vi "CSMStandApp.vi"() -> ()   [LabVIEW 2020]
doc: "------------- lvcsm -------------\n[CSMStates]\nItem 0 = \"Event Structure\"\nItem 1 = \"Idle\"\nItem 2 = \"CSM Documentation\"\nItem 3 = \"VI Reference\"\nItem 4 = \"Error Handler\"\nItem 5 = \"Critical Error\"\nItem 6 = \"Target Timeout Error\"\nItem 7 = \"Target Error\"\nItem 8 = \"Async Response\"\nItem 9 = \"Response\"\nItem 10 = \"Async Message Posted\"\nItem 11 = \"Initialize Core Data\"\nItem 12 = \"Exit\"\nItem 13 = \"Data: Initialize\"\nItem 14 = \"Data: Get Configuration\"\nItem 15 = \"Data: Get Internal Data\"\nItem 16 = \"Data: Set Configuration\"\nItem 17 = \"Data: Cleanup\"\nItem 18 = \"Events: Register\"\nItem 19 = \"Events: Unregister\"\nItem 20 = \"UI: Initialize\"\nItem 21 = \"UI: Cursor Set\"\nItem 22 = \"UI: Front Panel State\"\nItem 23 = \"UI: Insert CSMStand OI\"\nItem 24 = \"UI: Start CSMStand Engine Behind\"\nItem 25 = \"UI: Show Version Dialog\"\nItem 26 = \"UI: Update Title\"\nItem 27 = \"Macro: Initialize\"\nItem 28 = \"Macro: Exit\"\nItem 29 = \"API: Load Script File\"\nItem 30 = \"API: Information\"\nItem 31 = \"API: Settings\"\nItem 32 = \"Action: Action1\"\nItem 33 = \"Action: Action2\"\n\n[CSMStatus]\nItem 0 = \"Error Occurred@Error Handler\""
uses:
  f71e1bc3-10f1-4d1d-8987-c57c60744672.vi
  5479b9e0-3b99-47d2-9fb2-6b1a6c6fc50e.vi
  48aabd89-37f9-4145-9c04-d0fd28b441f4.vi
  35608a63-0d23-4e3c-87b1-9318b6aa47ba.vi
  c99d3ec9-4fb3-4a08-94ab-237d2d67cb16.vi
  b47ea106-f0ab-4a9d-a620-ab9fd917edd8.vi
  <userlib>/_NEVSTOP/Communicable State Machine(CSM)/AdvanceAPI/CSM - Revert Arguments-Safe String.vi
  <userlib>/_NEVSTOP/Communicable State Machine(CSM)/AdvanceAPI/CSM - Break Down Multiple States String.vi
  <userlib>/_NEVSTOP/Communicable State Machine(CSM)/AdvanceAPI/CSM - Compact Multiple States.vi
  <userlib>/_NEVSTOP/Communicable State Machine(CSM)/AdvanceAPI/CSM - Keywords.vi
  <userlib>/_NEVSTOP/Communicable State Machine(CSM)/_Shared/Trim Single-line Text.vi
  <userlib>/_NEVSTOP/Communicable State Machine(CSM)/addons/API-String-Arugments-Support/_Support/Query Data as API String Arguments(variant).vi
  <userlib>/_NEVSTOP/Communicable State Machine(CSM)/addons/API-String-Arugments-Support/_Support/Convert API String Arguments to Data(variant).vi
  CSMStand(Lite)/src/UI/ExecutionView(CSM).vi
  CSMStand(Lite)/src/Engine/Engine(CSM).vi
  CSMStand(Lite)/src/UI/VersionDialog(CSM).vi
  <userlib>/NEVSTOP-Programming-Palette/Dialog & Interface/Fit VI window to Visible Content_nevstop.vi
  <userlib>/NEVSTOP-Programming-Palette/Dialog & Interface/Fit VI window to Caller Center_nevstop.vi
  <userlib>/_NEVSTOP/Communicable State Machine(CSM)/addons/API-String-Arugments-Support/_Support/Data To API String Arguments.vi
  <userlib>/_NEVSTOP/Communicable State Machine(CSM)/addons/MassData-Parameter/_support/FGV-MassData(lvlibp).vi
  <userlib>/_NEVSTOP/Communicable State Machine(CSM)/Communicable State Machine.lvlib
  CSMStand(Lite)/CSMStand(Lite).lvlib
  <userlib>/_NEVSTOP/Communicable State Machine(CSM)/_tool/_ui/csm-ui-support.lvlib
  <userlib>/_NEVSTOP/Communicable State Machine(CSM)/addons/API-String-Arugments-Support/API String Arguments Support.lvlib
  <userlib>/_NEVSTOP/Communicable State Machine(CSM)/_tool/_file/csm-file-support.lvlib
  <userlib>/_NEVSTOP/Communicable State Machine(CSM)/_Shared/CSM Shared.lvlib
panel:
  in  "Toolbar.Information":bool
  in  "Toolbar.Load Script File":bool
  in  "Toolbar.Terminate":bool
  in  "Toolbar.SinglePass":bool
  out "Waveform Chart":dbl[](graph)
  out "LOG":string
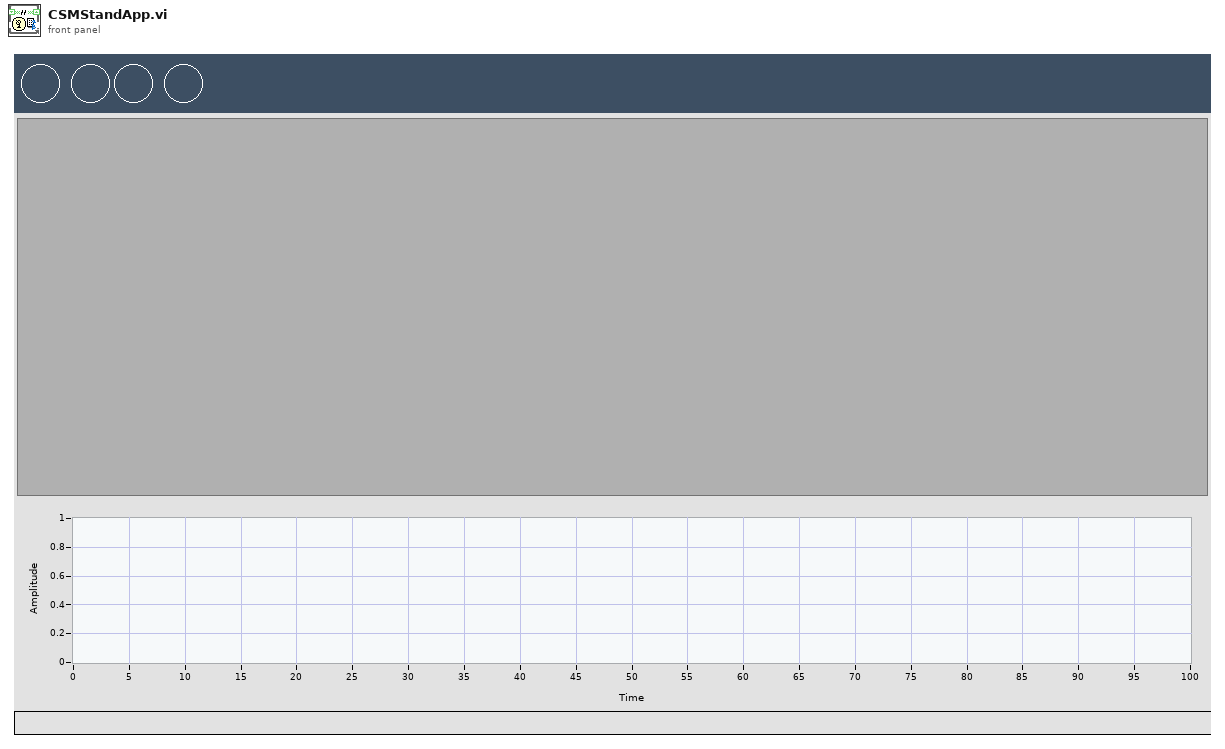
[diagram p1: front panel]
types:
  T1 = enum32{"Invalid", "Standard", "Closed", "Hidden", "Minimized", "Maximized"}
  T2 = enum32{"invalid app kind", "Development System", "Run Time System", "Student Edition", "Embedded LabVIEW", "Evaluation", "Custom"}
  T3 = typedef "Communicable State Machine.lvlib/_CSM_Response Source Message.ctl" = cluster{"‘State":string, "’Arguments":string, "’Error":errorcluster}
  T4 = cluster{"Current VI Reference":refnum<vi>, "Close Panel on Exit?":bool}
  T5 = cluster{"Core":cluster{"Current VI Reference":refnum<vi>, "Close Panel on Exit?":bool}, "DataBool":bool, "DataString":string, "Settings":cluster{"Boolean":bool, "string":string}}
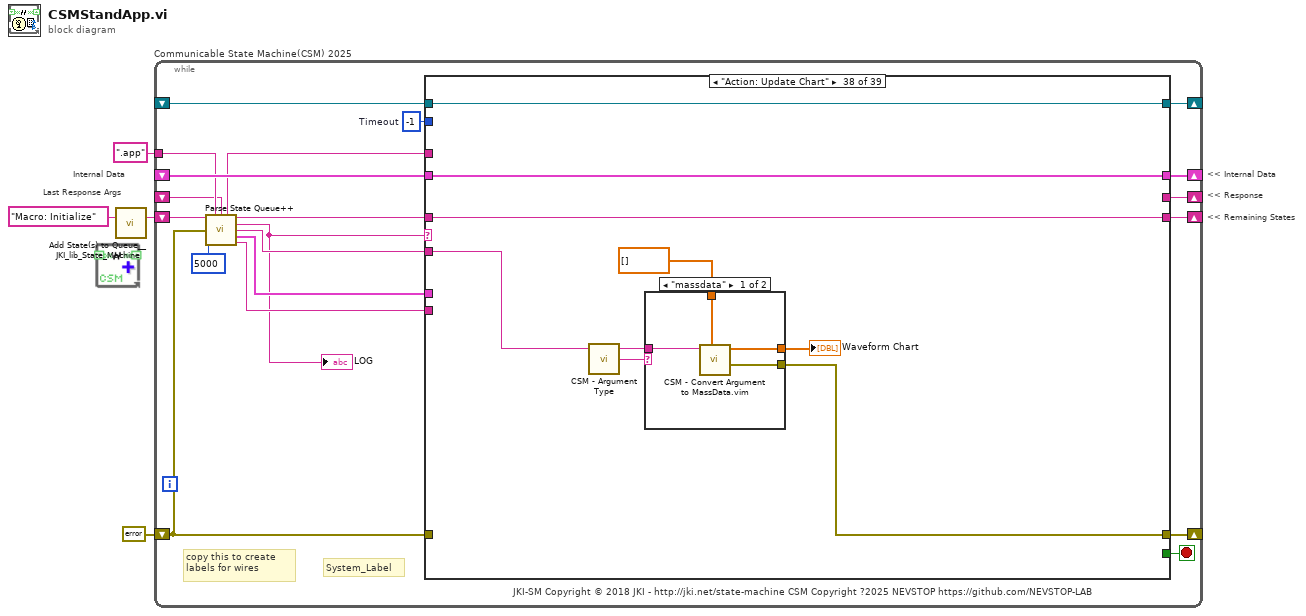
[diagram p0: block diagram]
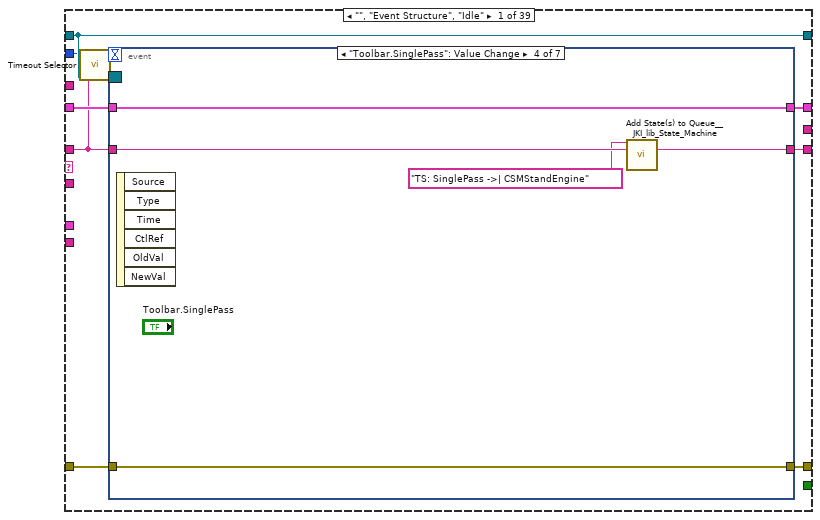
[diagram p2: hidden frame]
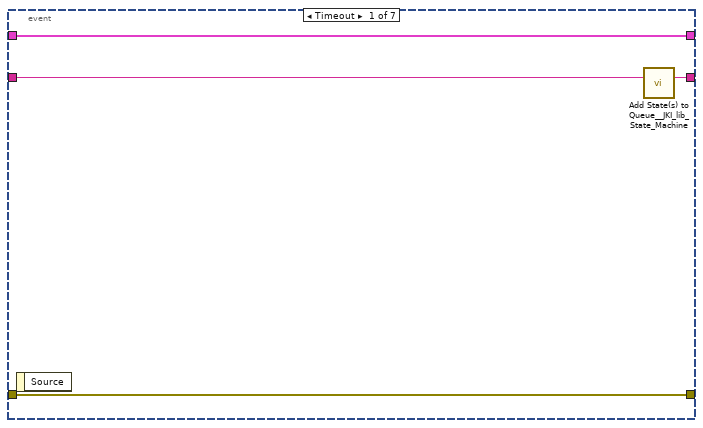
[diagram p3: hidden frame]
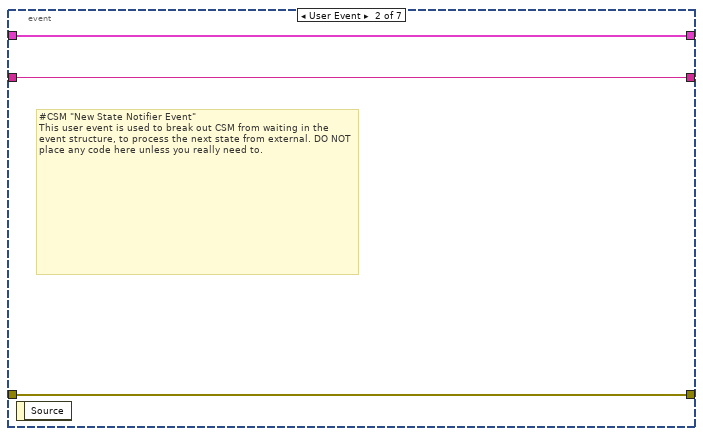
[diagram p4: hidden frame]
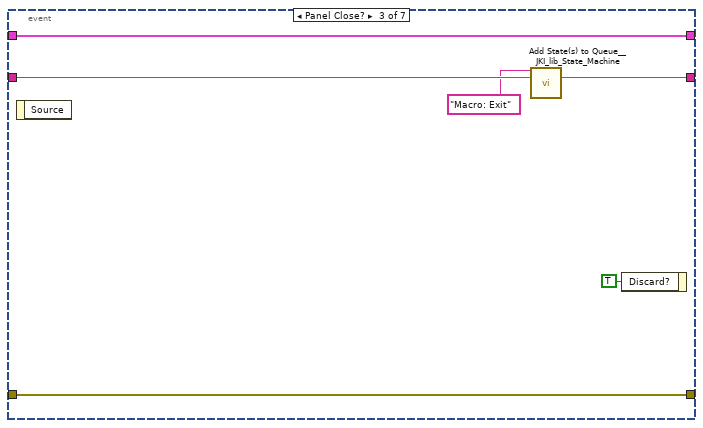
[diagram p5: hidden frame]
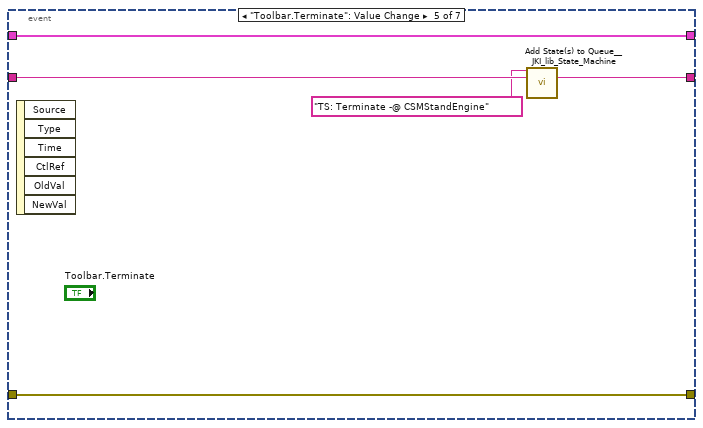
[diagram p6: hidden frame]
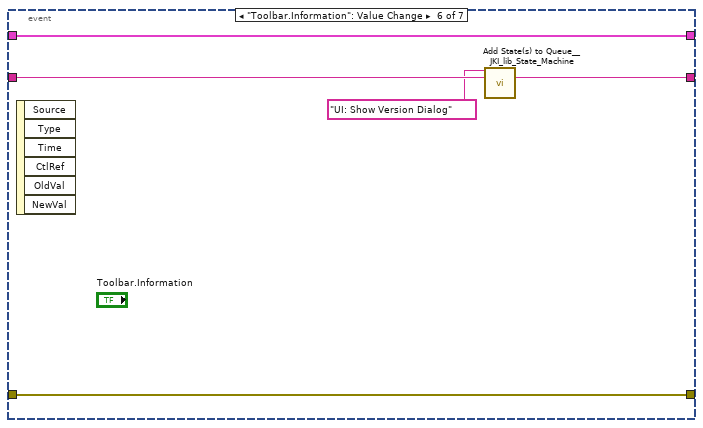
[diagram p7: hidden frame]
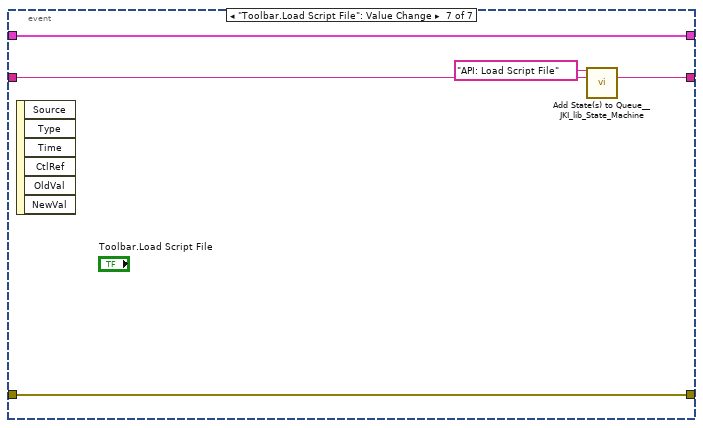
[diagram p8: hidden frame]
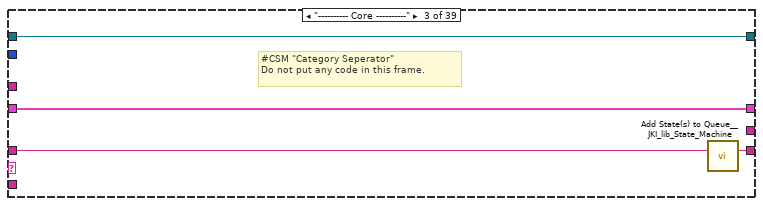
[diagram p10: hidden frame]
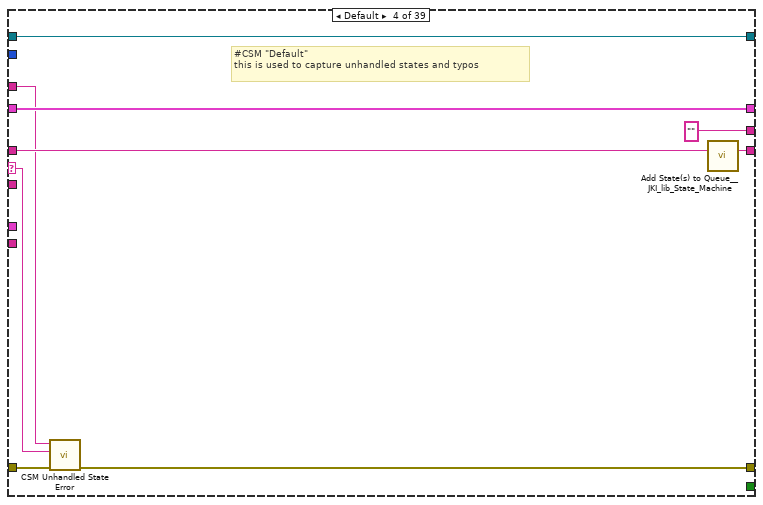
[diagram p11: hidden frame]
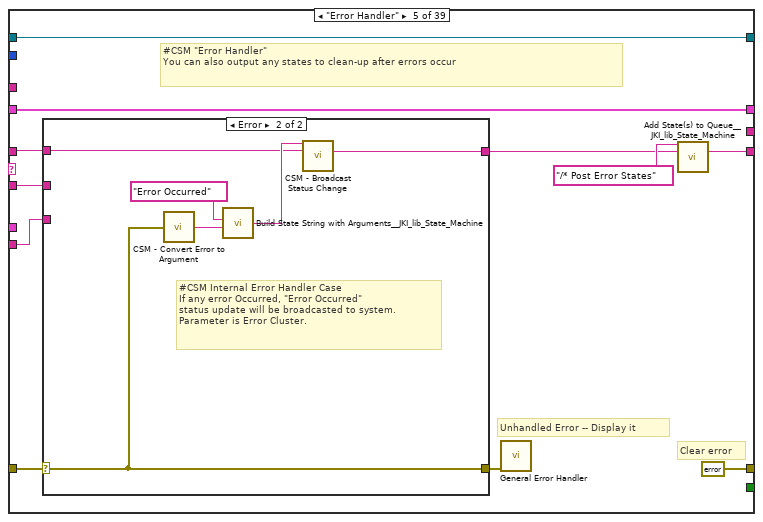
[diagram p12: hidden frame]
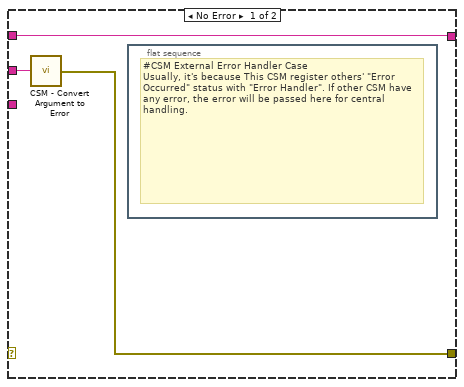
[diagram p13: hidden frame]
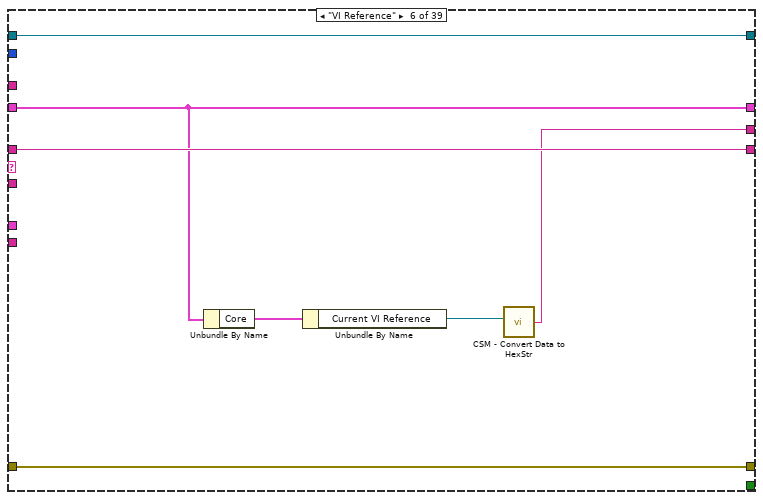
[diagram p14: hidden frame]
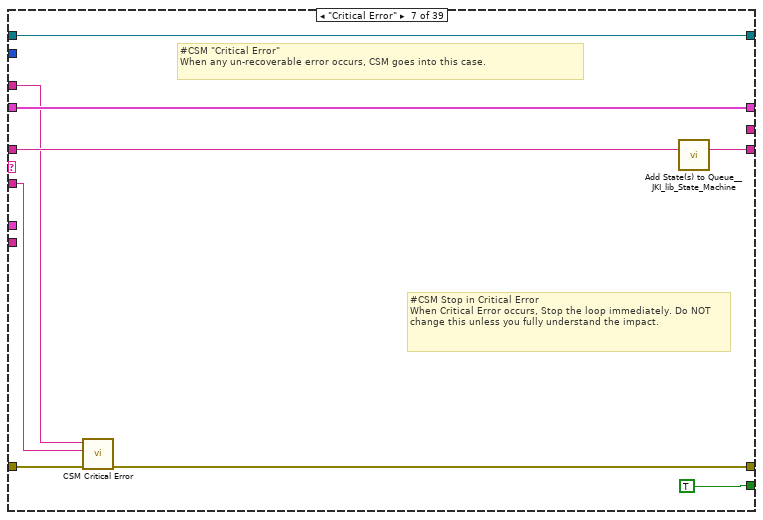
[diagram p15: hidden frame]
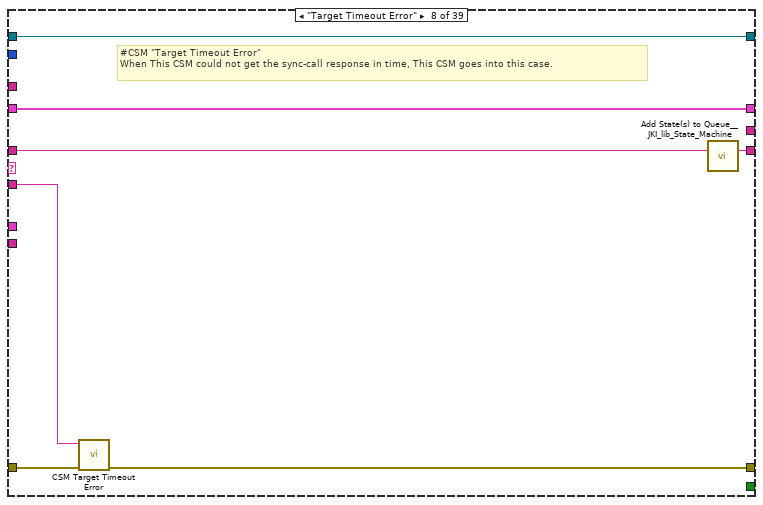
[diagram p16: hidden frame]
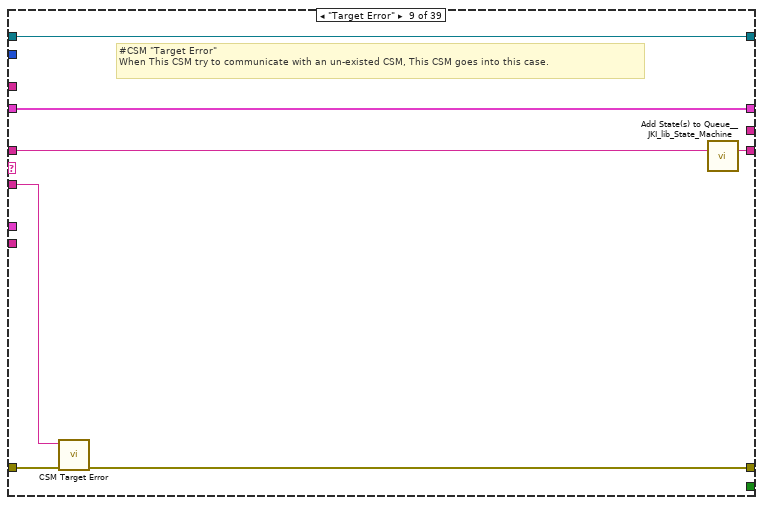
[diagram p17: hidden frame]
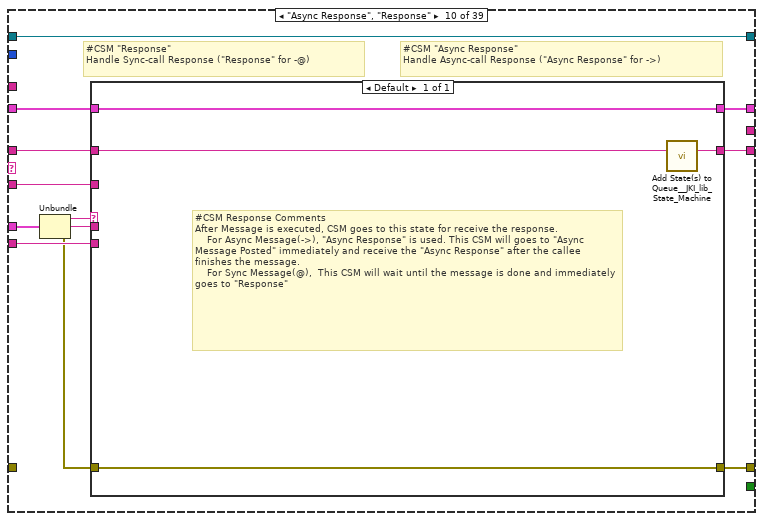
[diagram p18: hidden frame]
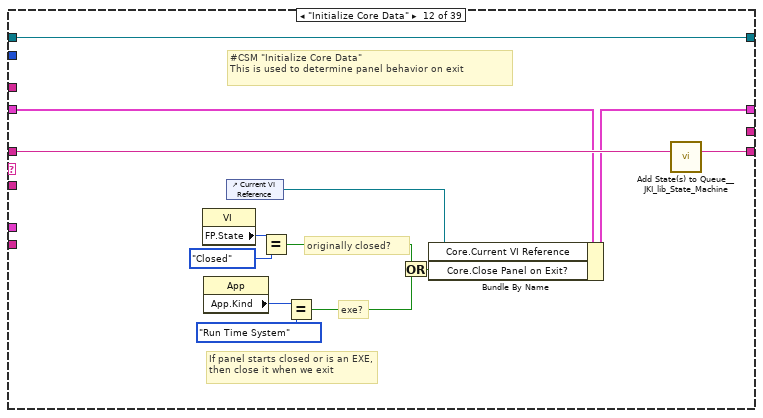
[diagram p20: hidden frame]
diagram:
  # "Last Response Args"
  # "Internal Data"
  # "<< Internal Data"
  # "<< Response"
  # "<< Remaining States"
  n1 = call <vilib>:"Add State(s) to Queue__JKI_lib_State_Machine.vi"("State(s) in (\"\")"="Macro: Initialize" ("Init States(\"Macro: Initialize\")")) -> ("States Out"=w3:string)  [unwired: 14 in]
  n2 = while "Communicable State Machine(CSM) 2025" {
    shift-right: [w19] -> _
    shift-left: _ -> [w18]
    shift-right: [w22] -> _
    shift-left: errorcluster {"status"=FALSE, "code"=0, "source"=""} ("error out") -> [w16]
    shift-right: [w21] -> _
    shift-left: w3 -> [w23]
    tunnel: ".app" ("Name(\"\" to use uuid)") -> [w11]
    shift-right: [w14] -> _
    shift-left: _ -> [w7]
    shift-right: [w13] -> _
    shift-left: _ -> [w12]
    stop <- w20 stop-if-true
    w17 = -1  # Timeout
    # "copy this to create labels for wires"
    # "System_Label"
    # "JKI-SM Copyright © 2018 JKI - http://jki.net/state-machine CSM Copyright ?2025 NEVSTOP https://github.com/NEVSTOP-LAB"
    n3 = call <userlib>:"Parse State Queue++.vi"("State Queue"=w23, "Name (\"\" to Use UUID)"=w11, "Response Arguments"=w7, "Previous Error"=w16, "Response Timeout (-2 Use Global Settings)"=5000 ("Response Timeout(1000ms)")) -> ("Name Used"=w8:string, "Remaining States"=w24:string, "Current State"=w5:string, "Arguments"=w6:string, ">> Response Source Message >>"=w10:T3, ">> Source CSM >>"=w9:string)  [unwired: 5 in]
    "LOG" <- w5
    n4 = case shown="\"Action: Update Chart\"" w5 {
      selector: w5 -> [_ _ _ w77 _ _ _ _ _ _ _ _ _ _ _ _ _ _ _ _ _ _ _ _ _ _ _ _ _ _ _ _ _ _ _ _ _ _ _]
      tunnel: w24 -> [w25 w69 w73 w80 w86 w108 w117 w124 w131 w137 w151 w164 w170 w174 w182 w189 w195 w201 w205 w212 w216 w220 w231 w238 w253 w331 w345 w366 w378 w383 w388 w404 w407 w413 w430 w433 w437 w446 w458]
      tunnel: w6 -> [_ _ _ _ w84 _ w115 w121 w128 w138 _ _ _ _ _ w184 w193 _ _ _ _ _ _ w233 w248 w315 w332 _ w371 _ _ _ _ _ _ _ _ w443 _]
      tunnel: w18 -> [w32 w68 w71 w78 w92 w104 w118 w122 w129 w136 w150 w158 w168 w172 _ w187 w192 w197 w203 w211 w215 w218 w229 w236 w250 w330 w344 w349 w376 w381 w386 w401 w406 w425 w429 w432 w435 w445 w457]
      tunnel: [w31 _ _ w82 errorcluster {"status"=FALSE, "code"=0, "source"=""} ("error out") w109 w111 w119 w126 w141 _ _ w167 _ _ w185 w190 w198 _ w206 w214 _ _ w234 w251 w316 w333 w350 w379 _ _ w402 _ w415 _ _ _ w438 w459] -> w22
      tunnel: w16 -> [w30 _ _ w81 w90 w109 w112 w125 w132 _ _ _ w167 _ _ _ _ _ _ _ _ _ _ w235 _ _ _ _ w379 _ _ w402 _ _ _ _ _ _ w459]
      tunnel: [w33 w69 w72 w79 w88 w108 w116 w123 w130 w134 w151 w163 w169 w173 w181 w189 w195 w200 w204 w212 w216 w219 w230 w237 w252 w331 w345 w366 w378 w382 w387 w403 w407 w414 w430 w433 w436 w446 w458] -> w21
      tunnel: [_ _ _ _ _ _ TRUE _ _ _ _ _ TRUE _ _ _ _ _ _ _ _ _ _ _ _ _ _ _ _ _ _ _ _ _ _ _ _ _ _] -> w20
      tunnel: [w29 w68 w71 w78 w92 w104 w118 w122 w129 w135 w150 w162 w168 w172 w180 w183 w191 w197 w203 w211 w215 w218 w229 w236 w250 w330 w344 w349 w376 w381 w386 w401 w406 w425 w429 w432 w435 w445 w457] -> w19
      tunnel: w17 -> [w27 _ _ _ _ _ _ _ _ _ _ _ _ _ _ _ _ _ _ _ _ _ _ _ _ _ _ _ _ _ _ _ _ _ _ _ _ _ _]
      tunnel: w9 -> [_ _ _ _ w83 _ _ _ _ w139 _ _ _ _ _ _ _ _ _ _ _ _ _ _ _ _ _ _ _ _ _ _ _ _ _ _ _ _ _]
      tunnel: w10 -> [_ _ _ _ _ _ _ _ _ w140 _ _ _ _ _ _ _ _ _ _ _ _ _ _ _ _ _ _ _ _ _ _ _ _ _ _ _ _ _]
      tunnel: [_ _ _ "" _ w103 _ _ _ _ _ _ _ _ _ w186 _ _ _ _ _ _ _ _ _ _ _ _ _ _ _ _ _ _ _ _ _ _ _] -> w14
      tunnel: [w28 w67 w70 w75 w91 w107 w113 w120 w127 w144 w149 w152 w165 w171 w176 w188 w194 w196 w202 w210 w213 w217 w228 w232 w247 w329 w343 w365 w377 w380 w384 w394 w405 w424 w428 w431 w434 w444 w456] -> w13
      tunnel: w12 -> [w28 w67 w70 w75 w91 w107 w113 w120 w127 w144 w149 w152 w165 w171 w176 w188 w194 w196 w202 _ w213 w217 w228 w232 w247 w329 w343 w365 w377 w380 w384 w394 w405 w424 w428 w431 w434 w444 w456]
      tunnel: w8 -> [_ _ _ w74 _ _ w110 _ _ _ _ _ _ _ _ _ _ _ _ w209 _ _ _ _ _ _ _ _ _ _ _ w392 _ _ _ _ _ _ _]
      frame "", "Event Structure", "Idle" {
        n5 = call <userlib>:"Timeout Selector.vi"("Remaining States"=w25, "Timeout Expected"=w27) -> ("Timeout"=w26:i32)  [unwired: 5 in]
        n6 = event shown="[3] \"Toolbar.SinglePass\": Value Change" {
          selector: w28 -> [_ _ _ _ _ _ _]
          dyn-events: _ -> [_ _ _ _ _ _ _]
          timeout: w26 -> [_ _ _ _ _ _ _]
          tunnel: w25 -> [w37 w39 w46 w48 w53 w58 w63]
          tunnel: [w36 w39 w45 w49 w54 w59 w64] -> w33
          tunnel: w32 -> [w34 w40 w43 w50 w55 w60 w65]
          tunnel: [w35 w38 w44 w51 w56 w61 w66] -> w31
          tunnel: w30 -> [w35 w38 w44 w51 w56 w61 w66]
          tunnel: [w34 w40 w43 w50 w55 w60 w65] -> w29
          event Timeout {
            n7 = event-data() -> ()  [unwired: 1 in, 1 out]
            n8 = call <vilib>:"Add State(s) to Queue__JKI_lib_State_Machine.vi"("State(s) in (\"\")"=w37) -> ("States Out"=w36:string)  [unwired: 14 in]
          }
          event User Event {
            # "#CSM \"New State Notifier Event\"\nThis user event is used to break out CSM from waiting in the event structure, to process the next state from external. DO NOT place any code here unless you really need to."
            n9 = event-data() -> ()  [unwired: 1 in, 1 out]
          }
          event Panel Close? {
            n10 = event-data() -> ()  [unwired: 1 in, 1 out]
            n11 = call <vilib>:"Add State(s) to Queue__JKI_lib_State_Machine.vi"("State(s) in Front (\"\")"="Macro: Exit", "State(s) in (\"\")"=w46) -> ("States Out"=w45:string)  [unwired: 13 in]
            n12 = event-data("Discard?"=TRUE) -> ()  [unwired: 1 in, 1 out]
          }
          event "Toolbar.SinglePass": Value Change {
            n13 = event-data() -> ()  [unwired: 1 in, 6 out]
            n14 = call <vilib>:"Add State(s) to Queue__JKI_lib_State_Machine.vi"("State(s) in Front (\"\")"="TS: SinglePass ->| CSMStandEngine" ("State(s) in Front (\"\")"), "State(s) in (\"\")"=w48) -> ("States Out"=w49:string)  [unwired: 13 in]
          }
          event "Toolbar.Terminate": Value Change {
            n15 = event-data() -> ()  [unwired: 1 in, 6 out]
            n16 = call <vilib>:"Add State(s) to Queue__JKI_lib_State_Machine.vi"("State(s) in Front (\"\")"="TS: Terminate -@ CSMStandEngine" ("State(s) in Front (\"\")"), "State(s) in (\"\")"=w53) -> ("States Out"=w54:string)  [unwired: 13 in]
          }
          event "Toolbar.Information": Value Change {
            n17 = event-data() -> ()  [unwired: 1 in, 6 out]
            n18 = call <vilib>:"Add State(s) to Queue__JKI_lib_State_Machine.vi"("State(s) in Front (\"\")"="UI: Show Version Dialog" ("State(s) in Front (\"\")"), "State(s) in (\"\")"=w58) -> ("States Out"=w59:string)  [unwired: 13 in]
          }
          event "Toolbar.Load Script File": Value Change {
            n19 = event-data() -> ()  [unwired: 1 in, 6 out]
            n20 = call <vilib>:"Add State(s) to Queue__JKI_lib_State_Machine.vi"("State(s) in Front (\"\")"="API: Load Script File" ("State(s) in Front (\"\")"), "State(s) in (\"\")"=w63) -> ("States Out"=w64:string)  [unwired: 13 in]
          }
        }
      }
      frame "CSM Documentation" {
        # "#CSM State Syntax\n\n// Comment line, all text to the right of “//” will be ignored\n// Local Message Example\nDoSth: DoA >> Arguments\n\n// Sync Call Example\nAPI: xxxx >> Arguments -@ TargetModule\n\n// Async Call Example\nAPI: xxxx >> Arguments -> TargetModule\n\n// Async Call without Reply Example\nAPI: xxxx >> Arguments ->| TargetModule\n\n// Broadcast normal status:\nStatus >> StatusArguments  -><status>\n\n// Broadcast Interrupt status:\nInterrupt >> StatusArguments  -><interrupt>\n\n// Register Source Module's status to Handler Module\nStatus@Source Module >> Handler Module@Handler Module -><register>\n\n// Unegister Source Module's status\nStatus@Source Module >> Handler Module -><unregister>"
        # "#CSM README FIRST\n\nCommunicable State Machine(CSM) is a LabVIEW application framework that builds upon JKI State Machine(JKISM). It follows the pattern of JKISM and extends the keywords to describe message communication between modules, including concepts such as Sync-Message, Async-Message, Subscription/Unsubscription of status - essential elements for creating reusable code modules. For more information, please visit the CSM wiki: https://nevstop-lab.github.io/CSM-Wiki/\n\nFor instructions on JKI State Machine, visit: \n    http://jki.net/state-machine/\nFor information about CSM, visit: \n    https://github.com/NEVSTOP-LAB"
        # "#CSM \"Documentation\"\nCase for holding CSM Documenation"
      }
      frame "---------- Core ----------" {
        # "#CSM \"Category Seperator\"\nDo not put any code in this frame."
        n21 = call <vilib>:"Add State(s) to Queue__JKI_lib_State_Machine.vi"("State(s) in (\"\")"=w73) -> ("States Out"=w72:string)  [unwired: 14 in]
      }
      frame Default {
        # "#CSM \"Default\"\nthis is used to capture unhandled states and typos"
        n22 = call <userlib>:"CSM Unhandled State Error.vi"("error in (no error)"=w81, "Current State"=w77, "CSM Name"=w74) -> ("error out"=w82:errorcluster)  [unwired: 8 in]
        n23 = call <vilib>:"Add State(s) to Queue__JKI_lib_State_Machine.vi"("State(s) in (\"\")"=w80) -> ("States Out"=w79:string)  [unwired: 14 in]
      }
      frame "Error Handler" {
        # "Unhandled Error -- Display it"
        # "#CSM \"Error Handler\"\nYou can also output any states to clean-up after errors occur"
        # "Clear error"
        n24 = case shown="Error" w90 {
          selector: w90 -> [_ w97]
          tunnel: [w95 w99] -> w87
          tunnel: w86 -> [w95 w98]
          tunnel: [w94 w97] -> w85
          tunnel: w84 -> [w96 _]
          tunnel: w83 -> [_ _]
          frame No Error {
            n25 = call <userlib>:"CSM - Convert Argument to Error.vi"("Argument"=w96) -> ("Error"=w94:errorcluster)  [unwired: 4 in]
            n26 = flat-sequence {
              frame #0 {
                # "#CSM External Error Handler Case\nUsually, it's because This CSM register others' \"Error Occurred\" status with \"Error Handler\". If other CSM have any error, the error will be passed here for central handling."
              }
            }
          }
          frame Error {
            # "#CSM Internal Error Handler Case \nIf any error Occurred, \"Error Occurred\" \nstatus update will be broadcasted to system.\nParameter is Error Cluster."
            n27 = call <userlib>:"CSM - Convert Error to Argument.vi"("Error"=w97) -> ("Argument"=w101:string)  [unwired: 4 in]
            n28 = call <vilib>:"Build State String with Arguments__JKI_lib_State_Machine.vi"("Arguments (\"\")"=w101, "State"="Error Occurred" ("Status with Arguments")) -> ("State with Arguments"=w100:string)  [unwired: 4 in]
            n29 = call <userlib>:"CSM - Broadcast Status Change.vi"("Status With Arguments"=w100, "State Queue"=w98) -> ("Remaining States"=w99:string)  [unwired: 13 in]
          }
        }
        n30 = call <vilib>:"General Error Handler.vi"("error in (no error)"=w85) -> ()  [unwired: 10 in, 5 out]
        n31 = call <vilib>:"Add State(s) to Queue__JKI_lib_State_Machine.vi"("State(s) in Front (\"\")"="/* Post Error States", "State(s) in (\"\")"=w87) -> ("States Out"=w88:string)  [unwired: 13 in]
      }
      frame "VI Reference" {
        n32 = Unbundle By Name(w104) -> ("Core"=w106:T4)
        n33 = Unbundle By Name(w106) -> ("Current VI Reference"=w105:refnum<vi>)
        n34 = call <userlib>:"CSM - Convert Data to HexStr.vi"("Variant"=w105) -> ("HEX String (0-9,A-F)"=w103:string)  [unwired: 8 in]
      }
      frame "Critical Error" {
        # "#CSM \"Critical Error\"\nWhen any un-recoverable error occurs, CSM goes into this case."
        # "#CSM Stop in Critical Error\nWhen Critical Error occurs, Stop the loop immediately. Do NOT change this unless you fully understand the impact."
        n35 = call <userlib>:"CSM Critical Error.vi"("error in (no error)"=w112, "Arugments (As Reason)"=w115, "CSM Name"=w110) -> ("error out"=w111:errorcluster)  [unwired: 8 in]
        n36 = call <vilib>:"Add State(s) to Queue__JKI_lib_State_Machine.vi"("State(s) in (\"\")"=w117) -> ("States Out"=w116:string)  [unwired: 14 in]
      }
      frame "Target Timeout Error" {
        # "#CSM \"Target Timeout Error\"\nWhen This CSM could not get the sync-call response in time, This CSM goes into this case."
        n37 = call <userlib>:"CSM Target Timeout Error.vi"("error in (no error)"=w125, "Arguments (As CSM Name)"=w121) -> ("error out"=w119:errorcluster)  [unwired: 9 in]
        n38 = call <vilib>:"Add State(s) to Queue__JKI_lib_State_Machine.vi"("State(s) in (\"\")"=w124) -> ("States Out"=w123:string)  [unwired: 14 in]
      }
      frame "Target Error" {
        # "#CSM \"Target Error\"\nWhen This CSM try to communicate with an un-existed CSM, This CSM goes into this case."
        n39 = call <userlib>:"CSM Target Error.vi"("error in (no error)"=w132, "Arguments (As CSM Name)"=w128) -> ("error out"=w126:errorcluster)  [unwired: 9 in]
        n40 = call <vilib>:"Add State(s) to Queue__JKI_lib_State_Machine.vi"("State(s) in (\"\")"=w131) -> ("States Out"=w130:string)  [unwired: 14 in]
      }
      frame "Async Response", "Response" {
        # "#CSM \"Async Response\"\nHandle Async-call Response (\"Async Response\" for ->)"
        # "#CSM \"Response\"\nHandle Sync-call Response (\"Response\" for -@)"
        n41 = Unbundle(w140) -> ("‘State"=w143:string, "’Arguments"=w142:string, "’Error"=w133:errorcluster)
        n42 = case shown="Default" w143 {
          tunnel: [w145] -> w134
          tunnel: w137 -> [w146]
          tunnel: [w148] -> w135
          tunnel: w136 -> [w148]
          tunnel: [w147] -> w141
          tunnel: w133 -> [w147]
          tunnel: w139 -> [_]
          tunnel: w138 -> [_]
          tunnel: w142 -> [_]
          frame Default {
            # "#CSM Response Comments\nAfter Message is executed, CSM goes to this state for receive the response.\n    For Async Message(->), \"Async Response\" is used. This CSM will goes to \"Async Message Posted\" immediately and receive the \"Async Response\" after the callee finishes the message.\n    For Sync Message(@),  This CSM will wait until the message is done and immediately goes to \"Response\""
            n43 = call <vilib>:"Add State(s) to Queue__JKI_lib_State_Machine.vi"("State(s) in (\"\")"=w146) -> ("States Out"=w145:string)  [unwired: 14 in]
          }
        }
      }
      frame "Async Message Posted" {
        # "#CSM \"Async Message Posted\"\nAfter Async Message is posted (-> or ->| ), CSM goes to this state for post-action.\nYou can use Argument - State to tell which Async Message is called."
      }
      frame "Initialize Core Data" {
        # "#CSM \"Initialize Core Data\"\nThis is used to determine panel behavior on exit"
        # "originally closed?"
        # "exe?"
        # "If panel starts closed or is an EXE, then close it when we exit"
        n44 = property class="VI"() -> ("FP.State"=w155:T1)  [unwired: 2 in, 2 out]
        n45 = property class="App"() -> ("App.Kind"=w161:T2)  [unwired: 2 in, 2 out]
        n46 = control-ref of="Current VI Reference"() -> (w156:refnum<vi>)
        n47 = Equal?(x=w155, y=T1."Closed" ("Front Panel Window:State")) -> (x = y?=w153:bool)
        n48 = Equal?(x=w161, y=T2."Run Time System" ("Application:Kind")) -> (x = y?=w159:bool)
        n49 = Or(x=w153, y=w159) -> (x .or. y?=w157:bool)
        n50 = Bundle By Name(cluster=w158, "Core.Current VI Reference"=w156, "Core.Close Panel on Exit?"=w157) -> (w162:T5)
        n51 = call <vilib>:"Add State(s) to Queue__JKI_lib_State_Machine.vi"("State(s) in (\"\")"=w164) -> ("States Out"=w163:string)  [unwired: 14 in]
      }
      frame "Exit" {
        # "#CSM \"Exit\"\nCase for exiting the loop. No errors that occur here will be handled."
        n52 = call <vilib>:"Add State(s) to Queue__JKI_lib_State_Machine.vi"("State(s) in (\"\")"=w170) -> ("States Out"=w169:string)  [unwired: 14 in]
      }
      frame "---------- Data ----------" {
        # "#CSM \"Category Seperator\"\nDo not put any code in this frame."
        n53 = call <vilib>:"Add State(s) to Queue__JKI_lib_State_Machine.vi"("State(s) in (\"\")"=w174) -> ("States Out"=w173:string)  [unwired: 14 in]
      }
      frame "Data: Initialize" {
        w175 = cluster{"Boolean":bool, "string":string} {"Boolean"=TRUE, "string"=""}  # Settings
        w177 = T4 {"Current VI Reference"=refnum, "Close Panel on Exit?"=FALSE}  # Core
        w179 = TRUE  # DataBool
        w178 = ""  # DataString
        # "Expand Bundle to add new data elements to shift register data."
        # "Data names and types of shift register data are defined by this bundle."
        # "do not delete - used by framework"
        # "#CSM \"Data: Initialize\"\nInitialize the shift-register data, here.\n(data names are defined by what you wire into the bundle function)"
        n54 = Bundle("Core"=w177, "DataBool"=w179, "DataString"=w178, "Settings"=w175) -> (w180:T5)  [unwired: 1 in]
        n55 = call <vilib>:"Add State(s) to Queue__JKI_lib_State_Machine.vi"("State(s) in (\"\")"=w182) -> ("States Out"=w181:string)  [unwired: 14 in]
      }
      frame "Data: Get Configuration", "Data: Get Internal Data" {
        n56 = call "Query Data as API String Arguments.vim"("Setting Name"=w184, "Internal Data"=w187) -> ("error"=w185:errorcluster, "Setting as String"=w186:string, "Internal Data(dup)"=w183:T5)  [unwired: 7 in]
      }
      frame "Data: Set Configuration" {
        n57 = call "Convert API String Arguments to Data.vim"("Type"=w192, "String"=w193) -> ("error"=w190:errorcluster, "Data"=w191:T5)  [unwired: 6 in]
      }
      frame "Data: Cleanup" {
        # "#CSM \"Data: Cleanup\"\nCleanup any data and references, here.\n(this is called automatically, by the Macro: Exit)"
        n58 = Unbundle By Name(w197) -> ("Core.Current VI Reference"=w199:refnum<vi>)
        n59 = Close Reference(reference=w199) -> (error out=w198:errorcluster)  [unwired: 1 in]
        n60 = call <vilib>:"Add State(s) to Queue__JKI_lib_State_Machine.vi"("State(s) in (\"\")"=w201) -> ("States Out"=w200:string)  [unwired: 14 in]
      }
      frame "---------- Events ----------" {
        # "#CSM \"Category Seperator\"\nDo not put any code in this frame."
        n61 = call <vilib>:"Add State(s) to Queue__JKI_lib_State_Machine.vi"("State(s) in (\"\")"=w205) -> ("States Out"=w204:string)  [unwired: 14 in]
      }
      frame "Events: Register" {
        # "#CSM \"Events: Register\"\nRegister user event. New Message Event is registered to break CSM waiting in event structure by default."
        # "#CSM Register New Message Event\nRegister message event to break Waiting in Event structure."
        n62 = call <userlib>:"CSM - Get New State Notifier Event.vi"("Name (\"\" to Use UUID) In"=w209) -> ("error out"=w207:errorcluster, "New State Notifier Event"=w208:refnum<user-event>)  [unwired: 9 in]
        n63 = register-events(error in=w207, w208) -> (reference out=w210:refnum<event-registration>, error out=w206:errorcluster)  [unwired: 1 in]
      }
      frame "Events: Unregister" {
        # "#CSM \"Events: Unregister\"\nUnregister user event."
        n64 = Unregister For Events(event registration refnum=w213) -> (error out=w214:errorcluster)  [unwired: 1 in]
      }
      frame "---------- UI ----------" {
        # "#CSM \"Category Seperator\"\nDo not put any code in this frame."
        n65 = call <vilib>:"Add State(s) to Queue__JKI_lib_State_Machine.vi"("State(s) in (\"\")"=w220) -> ("States Out"=w219:string)  [unwired: 14 in]
      }
      frame "UI: Initialize" {
        # "#CSM \"UI: Initialize\"\nInitialize the User Interface, here.\n(this is called automatically, by the Macro: Init)"
        n66 = control-ref of="Toolbar.Load Script File"() -> (w223:refnum<vi>)
        n67 = control-ref of="Toolbar.Terminate"() -> (w224:refnum<vi>)
        n68 = control-ref of="Toolbar.SinglePass"() -> (w225:refnum<vi>)
        n69 = control-ref of="Toolbar.Information"() -> (w226:refnum<vi>)
        n70 = control-ref of="Splitter"() -> (w227:refnum<vi>)
        n71 = Build Array(w223, w224, w225, w226) -> (w222:refnum<vi>[])
        n72 = call <userlib>:"Relocate Splitter Posistion.vi"("Array"=w222, "Splitter in"=w227) -> ()  [unwired: 9 in, 1 out]
        n73 = call <vilib>:"Add State(s) to Queue__JKI_lib_State_Machine.vi"("State(s) in Front (\"\")"="UI: Update Title" ("State(s) in Front (\"\")"), "State(s) in (\"\")"=w231) -> ("States Out"=w230:string)  [unwired: 13 in]
      }
      frame "UI: Cursor Set" {
        # "Argument"
        # "#CSM \"UI: Cursor Set\"\nSet and Unset Cursor Busy.\n(Usage: \"UI: Cursor Set >> Busy|Idle\")"
        n74 = disable-structure shown="Default" {
          disable-tunnel: w235 -> [w241 w246]
          disable-tunnel: [w240 w246] -> w234
          disable-tunnel: w233 -> [w239 _]
          frame condition #0 (active) {
            n75 = case shown="\"Busy\"" w239 {
              tunnel: w241 -> [w243 w245]
              tunnel: [w242 w244] -> w240
              frame "Idle", Default {
                n76 = call <vilib>:"Unset Busy.vi"("error in (no error)"=w243) -> ("error out"=w242:errorcluster)  [unwired: 10 in]
              }
              frame "Busy" {
                n77 = call <vilib>:"Set Busy.vi"("error in (no error)"=w245) -> ("error out"=w244:errorcluster)  [unwired: 9 in, 1 out]
              }
            }
          }
          frame condition #1 {
          }
        }
        n78 = call <vilib>:"Add State(s) to Queue__JKI_lib_State_Machine.vi"("State(s) in (\"\")"=w238) -> ("States Out"=w237:string)  [unwired: 14 in]
      }
      frame "UI: Front Panel State" {
        # "Argument"
        # "#CSM \"UI: Front Panel State\"\nSet Front Panel Open or Closed\n(Usage: \"UI: Front Panel State >> Open|Close\")"
        n79 = Unbundle By Name(w250) -> ("Core.Current VI Reference"=w249:refnum<vi>)
        n80 = case shown="\"Minimize\", \"Minimized\"" w248 {
          tunnel: [w260 w273 w284 w296 w308] -> w251
          tunnel: w249 -> [w259 w271 w283 w295 w307]
          frame "Open", "Standard", Default {
            w254 = T1."Standard" ("State")
            n81 = property class="VI"(reference=w259) -> (reference out=w257:refnum<vi>, error out=w258:errorcluster, "FP.State"=w256:T1)  [unwired: 1 in]
            n82 = Not Equal?(x=w256, y=w254) -> (x != y?=w255:bool)
            n83 = case shown="True" w255 {
              tunnel: [w264 w266] -> w260
              tunnel: w258 -> [w263 w266]
              tunnel: w257 -> [w262 _]
              tunnel: w254 -> [w261 _]
              frame True {
                n84 = invoke class="VI" method="FP.Open"(reference=w262, error in=w263, "Activate"=TRUE, "State"=w261) -> (error out=w264:errorcluster)  [unwired: 1 in, 4 out]
              }
              frame False {
              }
            }
          }
          frame "Close", "Closed" {
            n85 = property class="VI"(reference=w271) -> (reference out=w270:refnum<vi>, error out=w272:errorcluster, "FP.State"=w268:T1)  [unwired: 1 in]
            n86 = Not Equal?(x=w268, y=T1."Closed" ("Front Panel Window:State")) -> (x != y?=w267:bool)
            n87 = case shown="True" w267 {
              tunnel: [w274 w277] -> w273
              tunnel: w272 -> [w274 w276]
              tunnel: w270 -> [_ w275]
              frame False {
              }
              frame True {
                n88 = invoke class="VI" method="FP.Close"(reference=w275, error in=w276) -> (error out=w277:errorcluster)  [unwired: 1 in, 2 out]
              }
            }
          }
          frame "Hidden", "Hide" {
            w278 = T1."Hidden" ("State")
            n89 = property class="VI"(reference=w283) -> (reference out=w281:refnum<vi>, error out=w282:errorcluster, "FP.State"=w280:T1)  [unwired: 1 in]
            n90 = Not Equal?(x=w280, y=w278) -> (x != y?=w279:bool)
            n91 = case shown="True" w279 {
              tunnel: [w288 w289] -> w284
              tunnel: w282 -> [w287 w289]
              tunnel: w281 -> [w286 _]
              tunnel: w278 -> [w285 _]
              frame True {
                n92 = invoke class="VI" method="FP.Open"(reference=w286, error in=w287, "State"=w285) -> (error out=w288:errorcluster)  [unwired: 2 in, 4 out]
              }
              frame False {
              }
            }
          }
          frame "Minimize", "Minimized" {
            w290 = T1."Minimized" ("State")
            n93 = property class="VI"(reference=w295) -> (reference out=w293:refnum<vi>, error out=w294:errorcluster, "FP.State"=w292:T1)  [unwired: 1 in]
            n94 = Not Equal?(x=w292, y=w290) -> (x != y?=w291:bool)
            n95 = case shown="False" w291 {
              tunnel: [w300 w301] -> w296
              tunnel: w294 -> [w299 w301]
              tunnel: w293 -> [w298 _]
              tunnel: w290 -> [w297 _]
              frame True {
                n96 = invoke class="VI" method="FP.Open"(reference=w298, error in=w299, "State"=w297) -> (error out=w300:errorcluster)  [unwired: 2 in, 4 out]
              }
              frame False {
              }
            }
          }
          frame "Maximize", "Maximized" {
            w302 = T1."Maximized" ("State")
            n97 = property class="VI"(reference=w307) -> (reference out=w305:refnum<vi>, error out=w306:errorcluster, "FP.State"=w304:T1)  [unwired: 1 in]
            n98 = Not Equal?(x=w304, y=w302) -> (x != y?=w303:bool)
            n99 = case shown="True" w303 {
              tunnel: [w312 w313] -> w308
              tunnel: w306 -> [w311 w313]
              tunnel: w305 -> [w310 _]
              tunnel: w302 -> [w309 _]
              frame True {
                n100 = invoke class="VI" method="FP.Open"(reference=w310, error in=w311, "State"=w309) -> (error out=w312:errorcluster)  [unwired: 2 in, 4 out]
              }
              frame False {
              }
            }
          }
        }
        n101 = call <vilib>:"Add State(s) to Queue__JKI_lib_State_Machine.vi"("State(s) in (\"\")"=w253) -> ("States Out"=w252:string)  [unwired: 14 in]
      }
      frame "UI: Insert CSMStand OI" {
        n102 = vi-ref "CSMStand(Lite).lvlib:ExecutionView(CSM).vi"() -> (w321:refnum<vi>)
        n103 = property class="VI (strict)"(reference=w321) -> (reference out=w325:refnum<vi>, error out=w323:errorcluster, "Path"=w322:path)  [unwired: 1 in]
        n104 = Open VI Reference(type specifier VI Refnum (for type only)=w325, vi path=w322, options=128, error in (no error)=w323) -> (vi reference=w324:refnum<vi>, error out=w320:errorcluster)  [unwired: 2 in]
        n105 = call-by-ref "Start Asynchronous Call"(reference=w324, error in=w320, "Name(\"\" to use uuid)"=w315) -> (reference out=w327:refnum<vi>, error out=w326:errorcluster)  [unwired: 11 in]
        n106 = Close Reference(reference=w327, error in (no error)=w326) -> (error out=w318:errorcluster)
        n107 = call <userlib>:"CSM - Module VI Reference.vi"("error in (no error)"=w318, "Force? (F)"=TRUE, "CSM Name"=w315) -> ("error out"=w319:errorcluster, "CSM Module VIRef"=w317:refnum<vi>)  [unwired: 7 in]
        n108 = invoke on="Sub Panel" class="SubPnl" method="Insert VI"(error in=w319, "VI Ref"=w317) -> (error out=w316:errorcluster)  [unwired: 2 in, 3 out]
      }
      frame "UI: Start CSMStand Engine Behind" {
        n109 = vi-ref "CSMStand(Lite).lvlib:Engine(CSM).vi"() -> (w335:refnum<vi>)
        n110 = property class="VI (strict)"(reference=w335) -> (reference out=w339:refnum<vi>, error out=w337:errorcluster, "Path"=w336:path)  [unwired: 1 in]
        n111 = Open VI Reference(type specifier VI Refnum (for type only)=w339, vi path=w336, options=128, error in (no error)=w337) -> (vi reference=w338:refnum<vi>, error out=w334:errorcluster)  [unwired: 2 in]
        n112 = call-by-ref "Start Asynchronous Call"(reference=w338, error in=w334, "Name(\"\" to use uuid)"=w332) -> (reference out=w341:refnum<vi>, error out=w340:errorcluster)  [unwired: 11 in]
        n113 = Close Reference(reference=w341, error in (no error)=w340) -> (error out=w333:errorcluster)
      }
      frame "UI: Show Version Dialog" {
        w348 = "UI.VersionDlg" ("Name(\"\" to use uuid)")
        n114 = vi-ref "CSMStand(Lite).lvlib:VersionDialog(CSM).vi"() -> (w357:refnum<vi>)
        n115 = property class="VI (strict)"(reference=w357) -> (reference out=w361:refnum<vi>, error out=w359:errorcluster, "Path"=w358:path)  [unwired: 1 in]
        n116 = Open VI Reference(type specifier VI Refnum (for type only)=w361, vi path=w358, options=128, error in (no error)=w359) -> (vi reference=w360:refnum<vi>, error out=w356:errorcluster)  [unwired: 2 in]
        n117 = Unbundle By Name(w349) -> ("Core.Current VI Reference"=w346:refnum<vi>)
        n118 = call-by-ref "Start Asynchronous Call"(reference=w360, error in=w356, "Name(\"\" to use uuid)"=w348) -> (reference out=w363:refnum<vi>, error out=w362:errorcluster)  [unwired: 11 in]
        n119 = Close Reference(reference=w363, error in (no error)=w362) -> (error out=w355:errorcluster)
        n120 = call <userlib>:"CSM - Module VI Reference.vi"("error in (no error)"=w355, "CSM Name"=w348) -> ("error out"=w354:errorcluster, "CSM Module VIRef"=w353:refnum<vi>)  [unwired: 8 in]
        n121 = call-poly <userlib>:"Fit VI window_nevstop.vi"("error in (no error)"=w354, "border spacing (2 px)"=10, "VI Ref (calling VI)"=w353) -> ("error out"=w351:errorcluster, "dup VI Ref"=w347:refnum<vi>)  [unwired: 3 in]
        n122 = call-poly <userlib>:"Fit VI window_nevstop.vi"("Error In"=w351, "Caller VI Refnum (Callee's Caller)"=w346, "VI Ref (calling VI)"=w347) -> ("Error Out"=w350:errorcluster)  [unwired: 3 in, 1 out]
      }
      frame "UI: Update Title" {
        n123 = Unbundle By Name(w376) -> ("Core.Current VI Reference"=w375:refnum<vi>)
        n124 = call "Convert API String Arguments to Data.vim"("Type"=path "", "String"=w371) -> ("Data"=w370:path)  [unwired: 6 in, 1 out]
        n125 = Path To String(path=w370) -> (string=w368:string)
        n126 = call <userlib>:"Concatenate Strings If not Empty_csm.vi"("String"=w368, "seperator(:)"=" - ", "prefix"="CSMStand-Lite" ("Front Panel Window:Title")) -> ("result"=w374:string)  [unwired: 2 in]
        n127 = property class="VI"(reference=w375, "Front Panel.Title"=w374) -> (error out=w367:errorcluster)  [unwired: 1 in, 1 out]
        n128 = call <vilib>:"Clear Errors.vi"("error in (no error)"=w367) -> ()  [unwired: 5 in, 2 out]
      }
      frame "---------- Macro ----------" {
        # "#CSM \"Category Seperator\"\nDo not put any code in this frame."
        n129 = call <vilib>:"Add State(s) to Queue__JKI_lib_State_Machine.vi"("State(s) in (\"\")"=w383) -> ("States Out"=w382:string)  [unwired: 14 in]
      }
      frame "Macro: Initialize" {
        w385 = "Data: Initialize\nInitialize Core Data\nEvents: Register\nUI: Initialize\nAction: Reset Chart\nUI: Front Panel State >> Open\n//Start UI & Engine\nUI: Insert CSMStand OI >> CSMStandOI\nUI: Start CSMStand Engine Behind >> CSMStandEngine\n//Connect UI With Engine\nSequenceLoaded Event@CSMStandEngine >>TS: Load Sequence @CSMStandOI -><register> \nTestStarted Event@CSMStandEngine >>TS: Test Started Handler @CSMStandOI -><register> \nStepComplete Event@CSMStandEngine >>TS: Step Complete Handler @CSMStandOI -><register> \nTestComplete Event@CSMStandEngine >>TS: Test Complete Handler @CSMStandOI -><register> \nTestTerminated Event@CSMStandEngine >>TS: Test Complete Handler @CSMStandOI -><register>\nStepStart Event@CSMStandEngine >>TS: Step Start Handler @CSMStandOI -><register> "  # Data: Initialize Initialize Core Data Events: Register UI: Initialize Action: Reset Chart UI: Front Panel State >> Open //Start UI & Engine UI: Insert CSMStand OI >> CSMStandOI UI: Start CSMStand Engine Behind >> CSMStandEngine //Connect UI With Engine SequenceLoaded Event@CSMStandEngine >>TS: Load Sequence @CSMStandOI -><register>  TestStarted Event@CSMStandEngine >>TS: Test Started Handler @CSMStandOI -><register>  StepComplete Event@CSMStandEngine >>TS: Step Complete Handler @CSMStandOI -><register>  TestComplete Event@CSMStandEngine >>TS: Test Complete Handler @CSMStandOI -><register>  TestTerminated Event@CSMStandEngine >>TS: Test Complete Handler @CSMStandOI -><register> StepStart Event@CSMStandEngine >>TS: Step Start Handler @CSMStandOI -><register>
        # "#CSM \"Macro: Initialize\"\nInitialization Macro (This is called once, when the VI starts)"
        n130 = call <vilib>:"Add State(s) to Queue__JKI_lib_State_Machine.vi"("State(s) in Front (\"\")"=w385, "State(s) in (\"\")"=w388) -> ("States Out"=w387:string)  [unwired: 13 in]
      }
      frame "Macro: Exit" {
        # "#CSM \"Macro: Exit\"\nExit Macro (This is called once, when the VI exits)"
        n131 = Unbundle By Name(w401) -> ("Core.Close Panel on Exit?"=w400:bool)
        n132 = call <userlib>:"CSM - List Modules.vi"() -> ("Module Names"=w391:string[])  [unwired: 10 in, 1 out]
        n133 = Search 1D Array(1D array=w391, element=w392) -> (index of element=w389:i32)  [unwired: 1 in]
        n134 = Delete From Array(array=w391, index=w389) -> (array with subset deleted=w390:string[])  [unwired: 1 in, 1 out]
        n135 = Select(t="UI: Front Panel State >> Close", s=w400, f="") -> (s? t:f=w397:string)
        n136 = call <userlib>:"CSM - Build Exit Messages of CSMs.vi"("CSMs"=w390) -> ("States"=w393:string)  [unwired: 14 in]
        n137 = call <vilib>:"Add State(s) to Queue__JKI_lib_State_Machine.vi"("State(s) in Front (\"\")"=w393, "State(s) in (\"\")"=w397, "State(s) at Back (\"\")"="Data: Cleanup\nEvents: Unregister\nExit") -> ("States Out"=w395:string)  [unwired: 12 in]
        n138 = call <vilib>:"Add State(s) to Queue__JKI_lib_State_Machine.vi"("State(s) in Front (\"\")"=w395, "State(s) in (\"\")"=w404) -> ("States Out"=w403:string)  [unwired: 13 in]
      }
      frame "---------- API ----------" {
        # "#CSM \"Category Seperator\"\nDo not put any code in this frame."
      }
      frame "API: Load Script File" {
        n139 = call "File Dialog"("pattern (all files)"="*.csmscript") -> ("selected path"=w409:path, "error out"=w422:errorcluster)  [unwired: 11 in, 2 out]
        n140 = Not A Number/Path/Refnum?(number/path/refnum=w409) -> (NaN/Path/Refnum?=w408:bool)
        n141 = call <userlib>:"TxtFile Load_CSM.vi"("error in (no error)"=w422, "Path"=w409) -> ("error out"=w416:errorcluster, "Text"=w421:string)  [unwired: 8 in]
        n142 = case shown="False" w408 {
          tunnel: [w427 _] -> w410
          tunnel: w409 -> [w426 _]
          frame False {
            n143 = call "Convert Data To API String Arguments.vim"("data"=w426) -> ("String"=w427:string)  [unwired: 7 in, 1 out]
          }
          frame True {
          }
        }
        n144 = call <vilib>:"Build State String with Arguments__JKI_lib_State_Machine.vi"("Arguments (\"\")"=w410, "State"="UI: Update Title" ("State(s) at Back (\"\")")) -> ("State with Arguments"=w412:string)  [unwired: 4 in]
        n145 = call <userlib>:"CSM - Make String Arguments Safe.vi"("Argument String"=w421) -> ("Safe Argument String"=w420:string)  [unwired: 8 in]
        n146 = call <userlib>:"CSM - Send Message and Wait for Reply.vi"("Error In (No Error)"=w416, "Target Module"="CSMStandEngine", "Arguments (\"\")"=w420, "State"="TS: Load Sequence") -> ("error out"=w418:errorcluster)  [unwired: 5 in, 2 out]
        n147 = call <vilib>:"Clear Errors.vi"("error in (no error)"=w418) -> ("error out"=w415:errorcluster)  [unwired: 5 in, 1 out]
        n148 = call <vilib>:"Add State(s) to Queue__JKI_lib_State_Machine.vi"("State(s) in (\"\")"=w413, "State(s) at Back (\"\")"=w412) -> ("States Out"=w414:string)  [unwired: 13 in]
      }
      frame "API: Information" {
      }
      frame "API: Settings" {
      }
      frame "---------- Action ----------" {
        # "#CSM \"Category Seperator\"\nDo not put any code in this frame."
        n149 = call <vilib>:"Add State(s) to Queue__JKI_lib_State_Machine.vi"("State(s) in (\"\")"=w437) -> ("States Out"=w436:string)  [unwired: 14 in]
      }
      frame "Action: Update Chart" {
        n150 = call <userlib>:"CSM - Argument Type.vi"("Arguments"=w443) -> ("Argument Type"=w439:string, "Arguments (Dup)"=w442:string)  [unwired: 3 in]
        n151 = case shown="\"massdata\"" w439 {
          tunnel: w442 -> [w450 w454]
          tunnel: dbl[] [] -> [w449 w453]
          tunnel: [w448 w452] -> w440
          tunnel: [w447 w451] -> w438
          frame "massdata" {
            n152 = call "CSM - Convert Argument to MassData.vim"("Type"=w449, "MassData Argument"=w450) -> ("error out"=w447:errorcluster, "Data"=w448:dbl[])  [unwired: 6 in]
          }
          frame Default {
            n153 = call "Convert API String Arguments to Data.vim"("Type"=w453, "String"=w454) -> ("error"=w451:errorcluster, "Data"=w452:dbl[])  [unwired: 6 in]
          }
        }
        "Waveform Chart" <- w440
      }
      frame "Action: Reset Chart" {
        n154 = property on="Waveform Chart" class="WFChart (strict)"("History Data"=dbl[] []) -> ()  [unwired: 2 in, 2 out]
      }
    }
  }
